vi "WriteAC-frequency.vi"(0 "LCRControl in":refnum<class "LCRControl.lvclass">, 1 "AC frequency [Hz]":i32, 3 "error in (no error)":errorcluster) -> (7 "LCRControl out":refnum<class "LCRControl.lvclass">, 10 "error out":errorcluster)   [LabVIEW 2018, in "LCRControl.lvclass"]
uses:
  LCRControl.lvclass
  LCRControl.lvclass/LCRControl.ctl
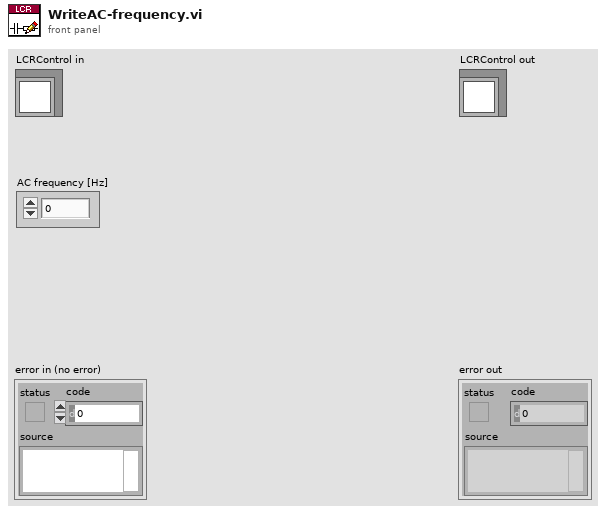
[diagram p1: front panel]
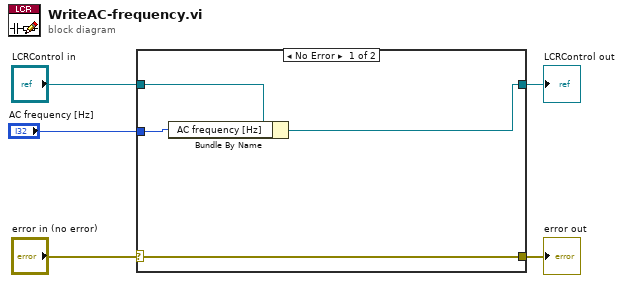
[diagram p0: block diagram]
diagram:
  n1 = case shown="No Error" "error in (no error)" {
    selector: "error in (no error)" -> [w9 w10]
    tunnel: [w9 w10] -> w4
    tunnel: [w7 w11] -> w2
    tunnel: "LCRControl in" -> [w8 w11]
    tunnel: "AC frequency [Hz]" -> [w6 _]
    frame No Error {
      n2 = Bundle By Name(cluster=w8, "AC frequency [Hz]"=w6) -> (w7:refnum<class "LCRControl.lvclass">)
    }
    frame Error {
    }
  }
  "error out" <- w4
  "LCRControl out" <- w2
